vi "GetStatus_EP.vi"(11 "Data":u8[](array[numeric])) -> (3 "Status":T1)   [LabVIEW 2014]
uses:
  Status_EP.ctl
panel:
  out "Boolean array":bool[][](array[boolean])
  out "Program change completed":bool
  out "Error clear Completed":bool
  out "Marking Completed":bool
  out "Marking Check NG":bool
  out "Marking Check OK":bool
  out "Marking Check Busy":bool
  out "Marking Check Score":u16
  out "Program Number":u16
  out "Marking Busy":bool
  out "Shutter":bool
  out "Warning":bool
  out "Error":bool
  out "Ready":bool
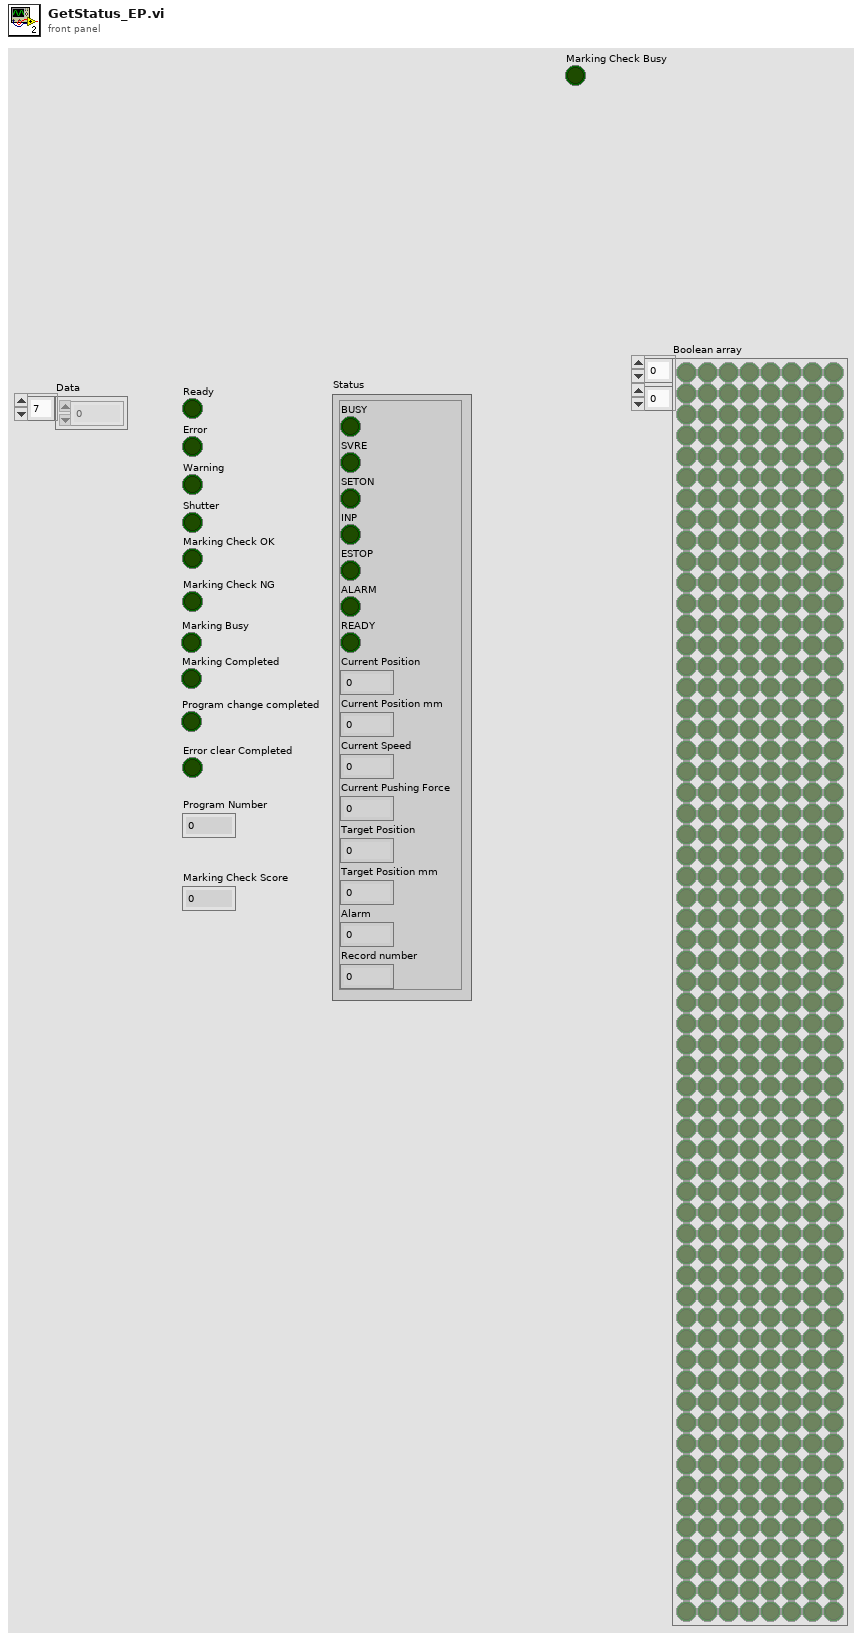
[diagram p1: front panel]
types:
  T1 = typedef "Status_EP.ctl" = cluster{"BUSY":bool, "SVRE":bool, "SETON":bool, "INP":bool, "ESTOP":bool, "ALARM":bool, "READY":bool, "Current Position":u32, "Current Position mm":dbl, "Current Speed":u16, "Current Pushing Force":u16, "Target Position":u32, "Target Position mm":dbl, "Alarm":u8, "Record number":u32}
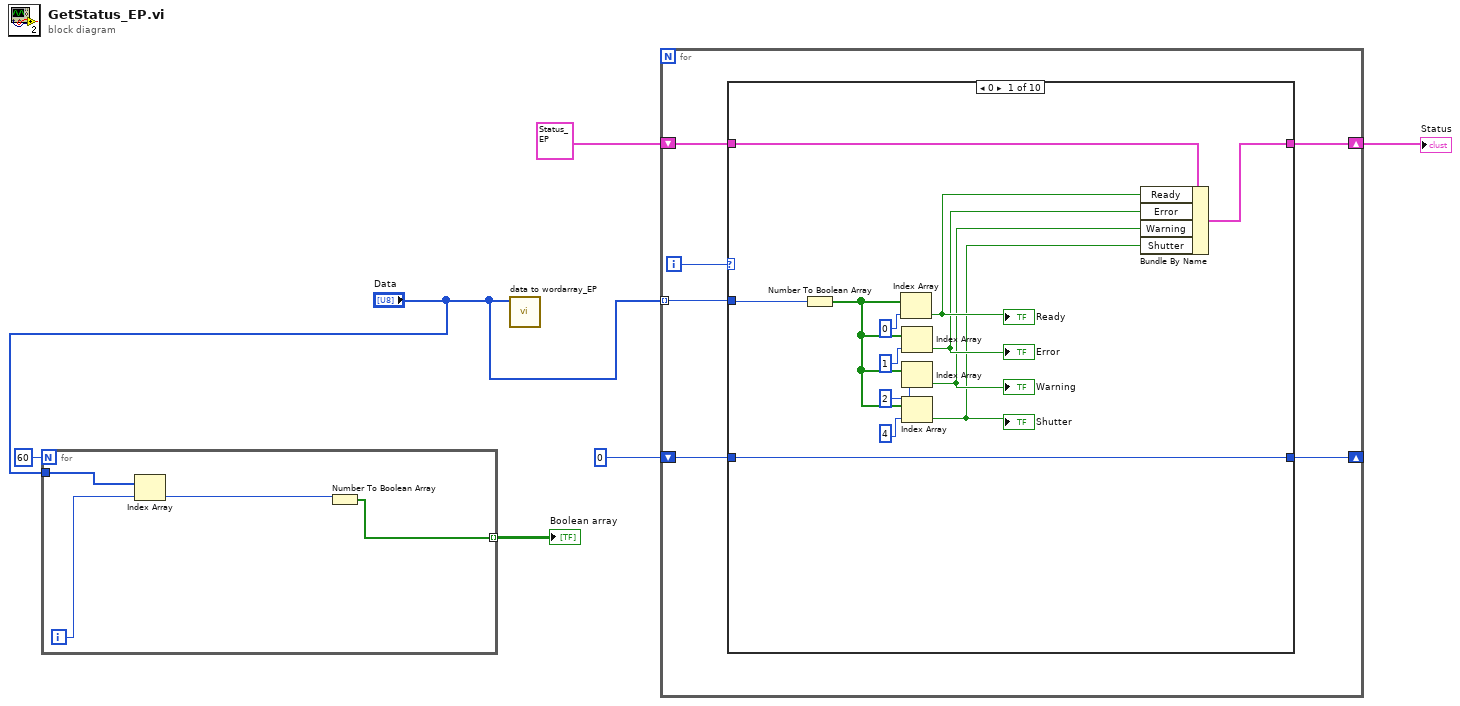
[diagram p0: block diagram]
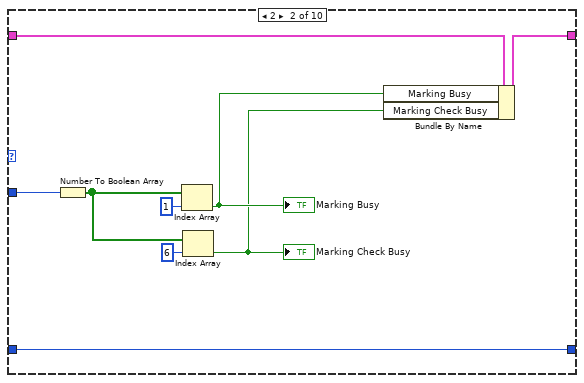
[diagram p2: hidden frame]
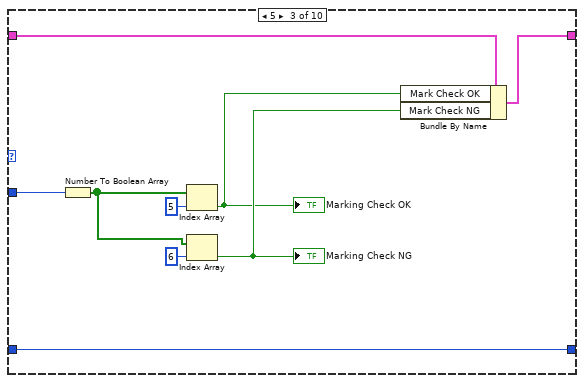
[diagram p3: hidden frame]
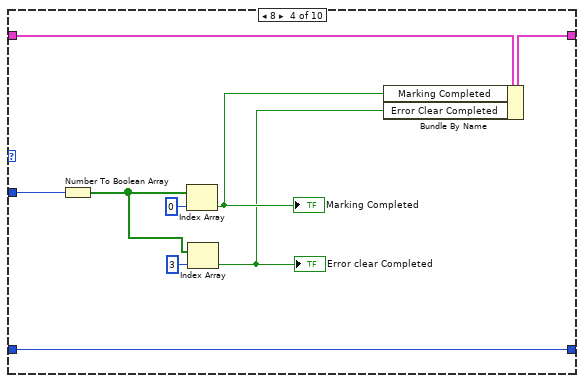
[diagram p4: hidden frame]
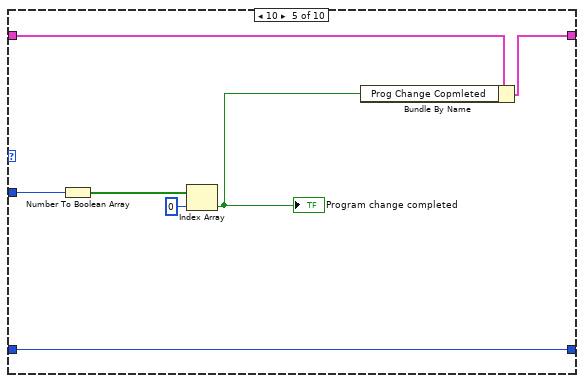
[diagram p5: hidden frame]
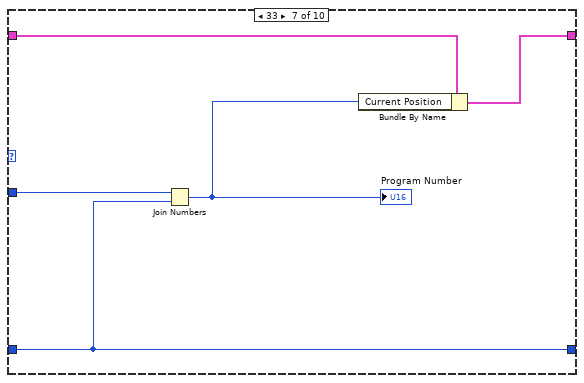
[diagram p7: hidden frame]
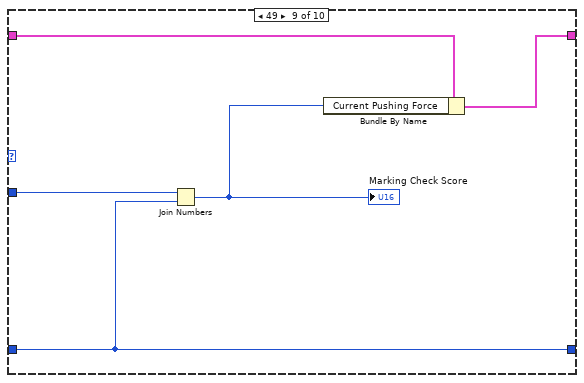
[diagram p9: hidden frame]
diagram:
  n1 = for {
    N: 60 -> [_]
    tunnel: "Data" -> [w10]
    tunnel: [w7] -> w2 mode=indexing
    i -> [w9]
    n2 = Index Array(array=w10, index=w9) -> (element=w8:u8)
    n3 = Number To Boolean Array(number=w8) -> (Boolean array=w7:bool[])
  }
  "Boolean array" <- w2
  n4 = call "data to wordarray_EP.vi"("Data"="Data") -> ()  [unwired: 10 in, 1 out]
  n5 = for {
    tunnel: "Data" -> [w15] mode=indexing
    shift-right: [w13] -> w5
    shift-left: T1 {"BUSY"=FALSE, "SVRE"=FALSE, "SETON"=FALSE, "INP"=FALSE, "ESTOP"=FALSE, "ALARM"=FALSE, "READY"=FALSE, "Current Position"=0, "Current Position mm"=0.0, "Current Speed"=0, "Current Pushing Force"=0, "Target Position"=0, "Target Position mm"=0.0, "Alarm"=0, "Record number"=0} ("Status") -> [w14]
    shift-right: [w11] -> _
    shift-left: i8 0 ("index") -> [w12]
    i -> [w16]
    n6 = case shown="0" w16 {
      tunnel: w15 -> [w19 w35 w41 w52 w59 w65 w68 w72 w75 _]
      tunnel: w14 -> [w25 w37 w43 w54 w61 w64 w70 w71 w77 w79]
      tunnel: [w24 w36 w42 w53 w60 w64 w69 w71 w76 w79] -> w13
      tunnel: w12 -> [w17 w30 w39 w48 w57 _ w66 _ w73 w78]
      tunnel: [w17 w30 w39 w48 w57 w65 w66 w72 w73 w78] -> w11
      frame 0 {
        n7 = Number To Boolean Array(number=w19) -> (Boolean array=w18:bool[])
        n8 = Index Array(array=w18, index=0) -> (element=w23:bool)
        "Ready" <- w23
        n9 = Index Array(array=w18, index=1) -> (element=w22:bool)
        "Error" <- w22
        n10 = Index Array(array=w18, index=2) -> (element=w21:bool)
        "Warning" <- w21
        n11 = Index Array(array=w18, index=4) -> (element=w20:bool)
        "Shutter" <- w20
        n12 = Bundle By Name(cluster=w25, "Ready"=w23, "Error"=w22, "Warning"=w21, "Shutter"=w20) -> (w24:T1)
      }
      frame 2 {
        n13 = Number To Boolean Array(number=w35) -> (Boolean array=w32:bool[])
        n14 = Index Array(array=w32, index=1) -> (element=w33:bool)
        "Marking Busy" <- w33
        n15 = Index Array(array=w32, index=6) -> (element=w31:bool)
        "Marking Check Busy" <- w31
        n16 = Bundle By Name(cluster=w37, "Marking Busy"=w33, "Marking Check Busy"=w31) -> (w36:T1)
      }
      frame 5 {
        n17 = Number To Boolean Array(number=w41) -> (Boolean array=w40:bool[])
        n18 = Index Array(array=w40, index=5) -> (element=w46:bool)
        "Marking Check OK" <- w46
        n19 = Index Array(array=w40, index=6) -> (element=w47:bool)
        "Marking Check NG" <- w47
        n20 = Bundle By Name(cluster=w43, "Mark Check OK"=w46, "Mark Check NG"=w47) -> (w42:T1)
      }
      frame 8 {
        n21 = Number To Boolean Array(number=w52) -> (Boolean array=w50:bool[])
        n22 = Index Array(array=w50, index=0) -> (element=w56:bool)
        "Marking Completed" <- w56
        n23 = Index Array(array=w50, index=3) -> (element=w49:bool)
        "Error clear Completed" <- w49
        n24 = Bundle By Name(cluster=w54, "Marking Completed"=w56, "Error Clear Completed"=w49) -> (w53:T1)
      }
      frame 10 {
        n25 = Number To Boolean Array(number=w59) -> (Boolean array=w58:bool[])
        n26 = Index Array(array=w58, index=0) -> (element=w63:bool)
        "Program change completed" <- w63
        n27 = Bundle By Name(cluster=w61, "Prog Change Copmleted"=w63) -> (w60:T1)
      }
      frame 32 {
      }
      frame 33 {
        n28 = Join Numbers(hi=w68, lo=w66) -> ((hi.lo)=w67:u16)
        "Program Number" <- w67
        n29 = Bundle By Name(cluster=w70, "Current Position"=w67) -> (w69:T1)
      }
      frame 48 {
      }
      frame 49 {
        n30 = Join Numbers(hi=w75, lo=w73) -> ((hi.lo)=w74:u16)
        "Marking Check Score" <- w74
        n31 = Bundle By Name(cluster=w77, "Current Pushing Force"=w74) -> (w76:T1)
      }
      frame Default {
      }
    }
  }
  "Status" <- w5
